vi "Sets_Intersect(STR).vi"(8 "error in (no error)":errorcluster caption="错误输入（无错误）", 10 "输入数组B":string[](array[string]), 11 "输入数组A":string[](array[string])) -> (0 "error out":errorcluster caption="错误输出", 3 "输出数组C":string[](array[string]))   [LabVIEW 2011]
uses:
  Sets_Unique(STR).vi
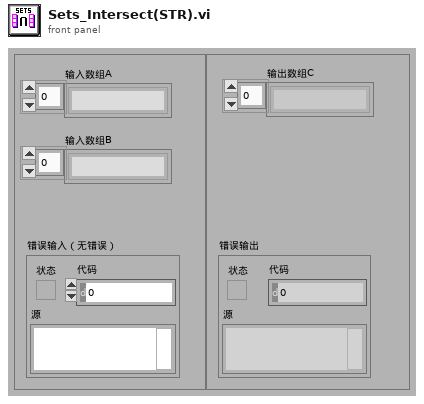
[diagram p1: front panel]
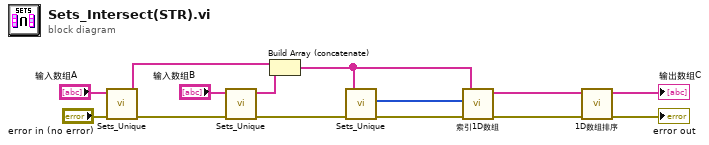
[diagram p0: block diagram]
diagram:
  n1 = call-poly "Sets_Unique.vi"("error in (no error)"="error in (no error)", "输入数组"="输入数组A") -> ("error out"=w11:errorcluster, "输出数组"=w3:string[])  [unwired: 7 in, 1 out]
  n2 = call-poly "Sets_Unique.vi"("error in (no error)"=w11, "输入数组"="输入数组B") -> ("error out"=w12:errorcluster, "输出数组"=w2:string[])  [unwired: 7 in, 1 out]
  n3 = Build Array (concatenate)(w3, w2) -> (w5:string[])
  n4 = call-poly "Sets_Unique.vi"("error in (no error)"=w12, "输入数组"=w5) -> ("error out"=w8:errorcluster, "已删除元素索引"=w6:i32[])  [unwired: 7 in, 1 out]
  n5 = call-poly "索引1D数组.vi"("error in (no error)"=w8, "索引"=w6, "输入数组"=w5) -> ("error out"=w7:errorcluster, "元素"=w1:string[])  [unwired: 7 in]
  n6 = call-poly "1D数组排序.vi"("error in (no error)"=w7, "输入数组"=w1) -> ("error out"=→"error out":errorcluster, "排序后数组"=→"输出数组C":string[])  [unwired: 7 in, 1 out]
